vi "myRIO_BRig_Host_v0,31.vi"() -> ()   [LabVIEW 2014]
panel:
  out "output_L_or_R":i32
  out "element":u16
  out "error_LoadPrevSettings":errorcluster caption="error out"
  in  "LoadPrevSettings":bool
  out "graph_ai1":dbl(graph)
  out "graph_ai0":dbl(graph)
  in  "dataIn_maxTrialsDisplayed":i32 caption="Number of Trials Displayed\n( 0 = all trials )"
  out "error_TCP":errorcluster
  in  "stop":bool
  in  "colorIn_timeout":u32(colorbox)=7468543 caption="Choice Timeout"
  in  "colorIn_wrong/cue":u32(colorbox)=16728618 caption="Wrong Choice or\nLicked During Cue"
  in  "colorIn_reward":u32(colorbox)=5898088 caption="Reward"
  in  "colorIn_unknown":u32(colorbox)=16449331 caption="Unknown Trial Status"
  out "dataOut_plot":cluster{i32[], i32[]}[](graph)
  out "iTrial":i32
  out "iBlock":i32
  # "Exp Stats"
  # "Current Block Stats"
  # "Trials 2 Reward\n\nBad Trials\nPost Reward"
  # "Left Spout    Right Spout"
  # "Run Time\n\n   minutes    seconds"
  # "Average Block Stats"
  # "Trials 2 Reward\n\nBad Trials\nPost Reward"
  # "Left Spout    Right Spout"
  # "If you get ERROR 5 related to opening a file, press CONTINUE"
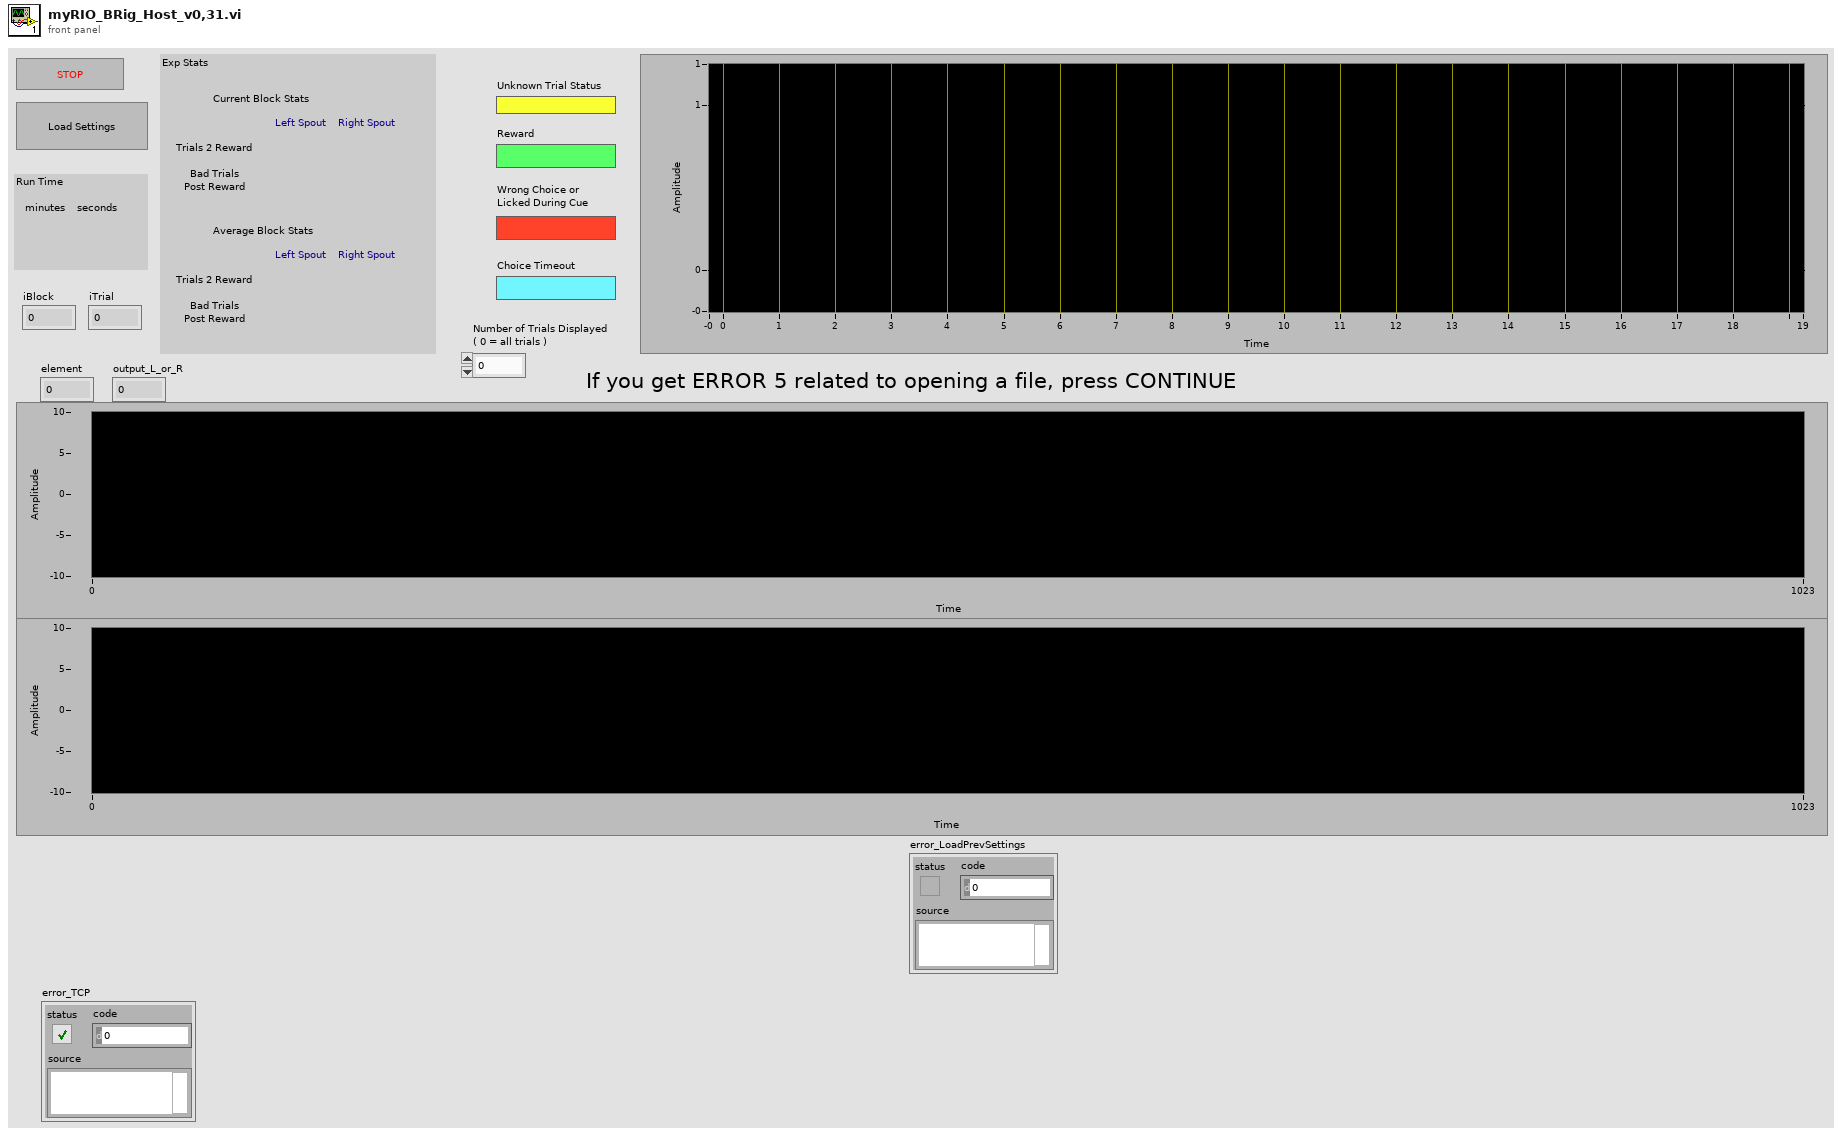
[diagram p1: front panel]
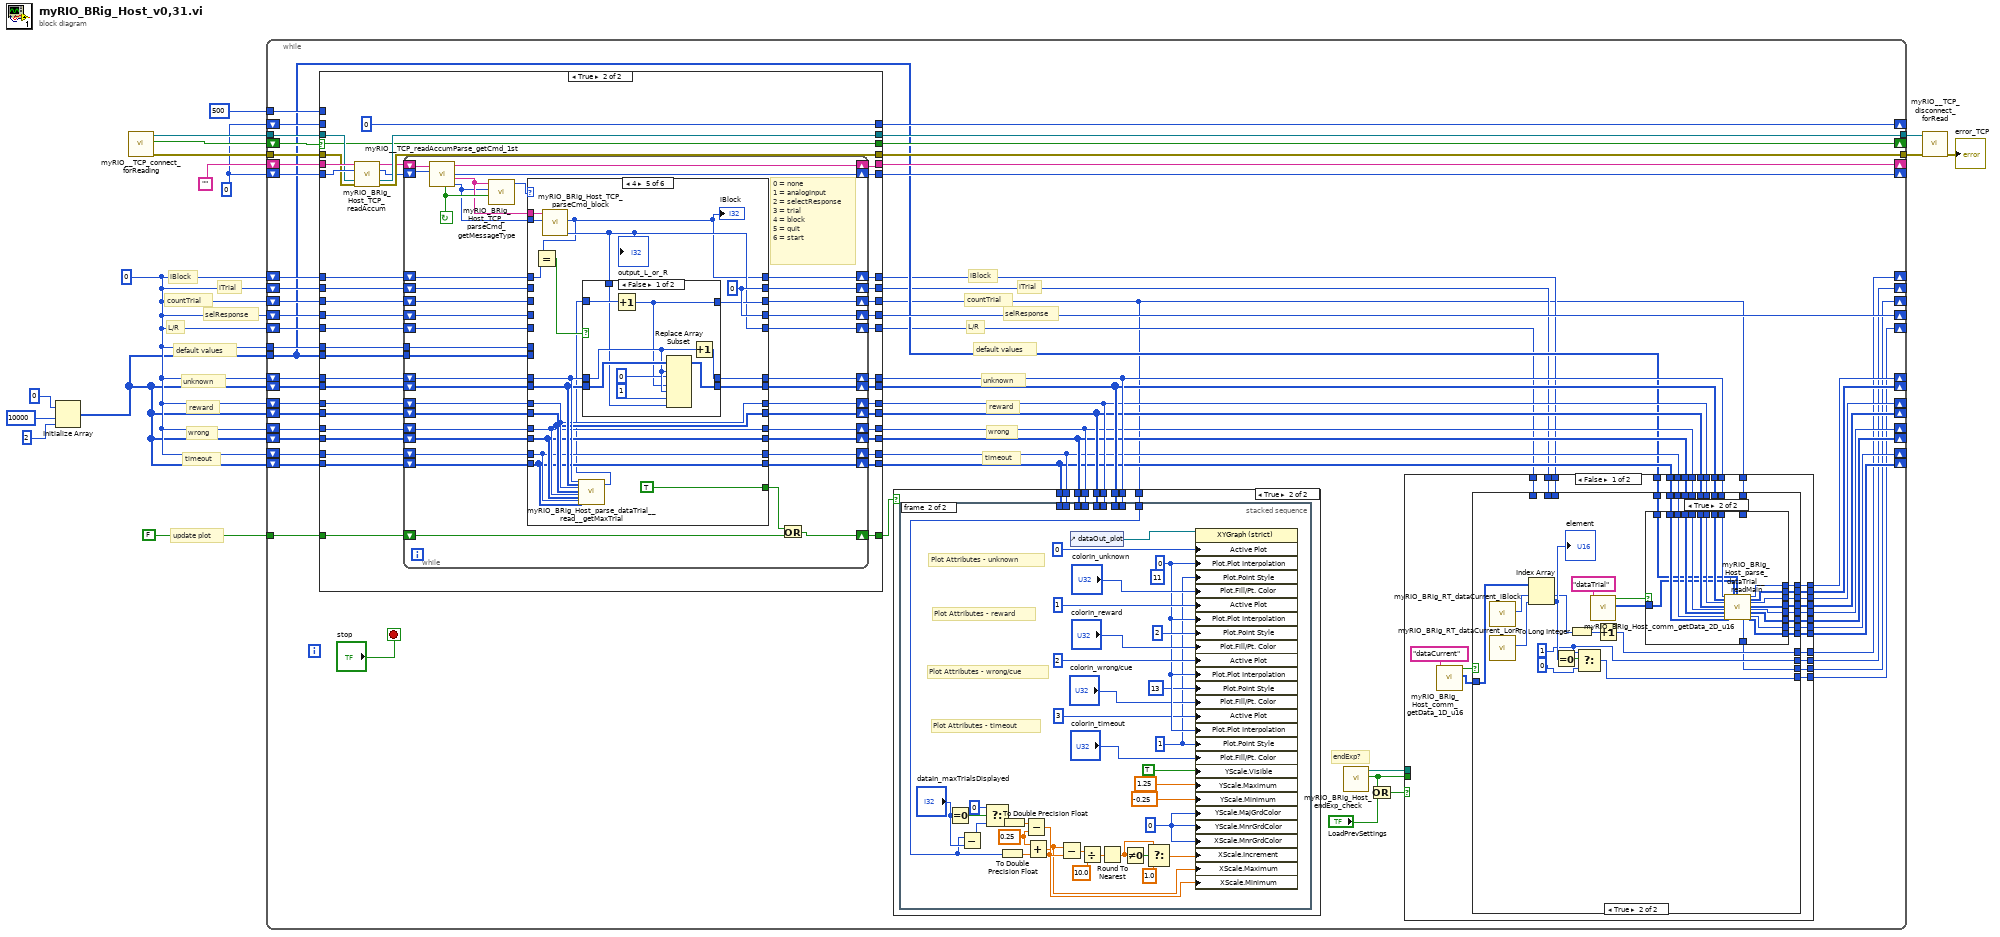
[diagram p0: block diagram]
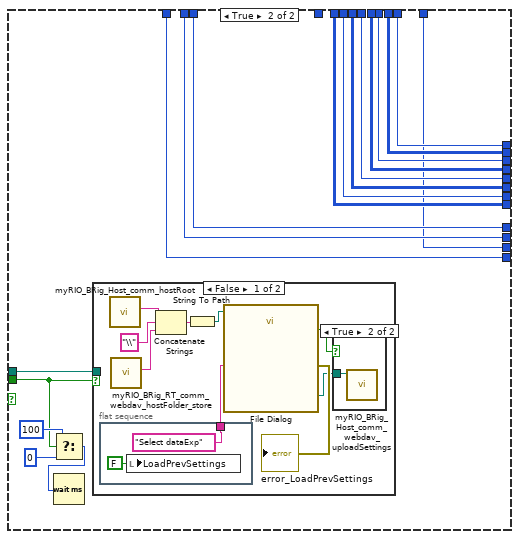
[diagram p4: hidden frame]
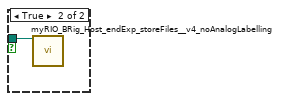
[diagram p6: hidden frame]
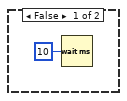
[diagram p7: hidden frame]
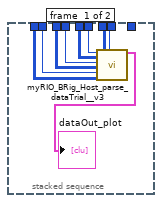
[diagram p8: hidden frame]
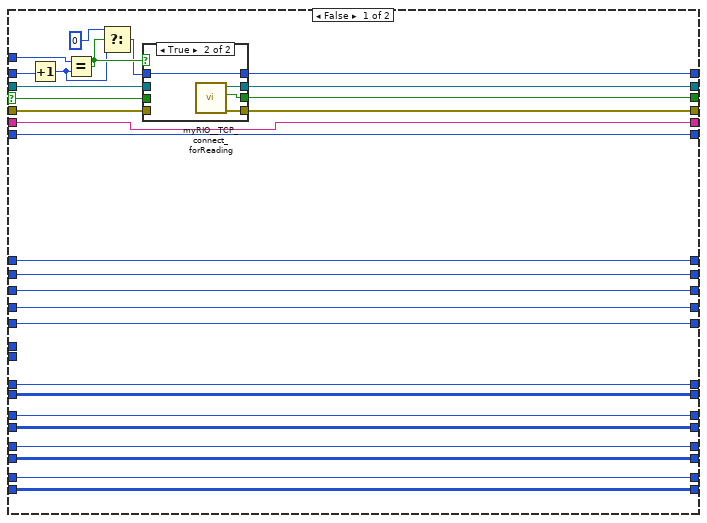
[diagram p9: hidden frame]
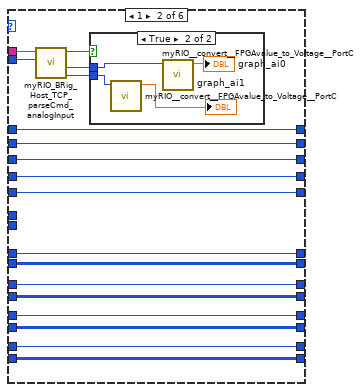
[diagram p12: hidden frame]
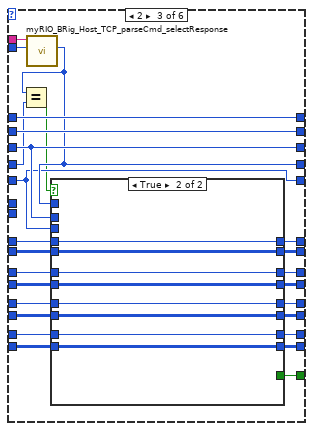
[diagram p14: hidden frame]
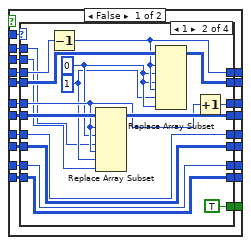
[diagram p15: hidden frame]
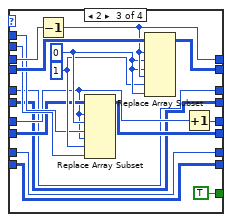
[diagram p17: hidden frame]
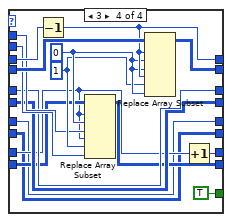
[diagram p18: hidden frame]
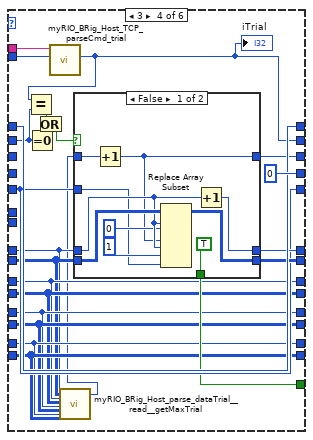
[diagram p19: hidden frame]
diagram:
  w2 = 0
  w11 = 0
  # "default values"
  # "update plot"
  # "timeout"
  # "wrong"
  # "reward"
  # "unknown"
  # "L/R"
  # "selResponse"
  # "countTrial"
  # "iBlock"
  # "iTrial"
  n1 = Initialize Array(0 ("element"), 10000 ("dimension size"), 2 ("dimension size")) -> (w1:i32[][])
  n2 = call "myRIO__TCP_connect_forReading.vi"() -> ("output_error"=w13:errorcluster, "output_connected"=w14:bool, "output_hTCP"=w15:refnum<k5>)  [unwired: 9 in]
  n3 = while {
    tunnel: w15 -> [w74]
    tunnel: w13 -> [w72]
    shift-right: [w65] -> _
    shift-left: w11 -> [w70]
    shift-right: [w66] -> _
    shift-left: "" -> [w71]
    shift-right: [w67] -> _
    shift-left: w14 -> [w73]
    shift-right: [w68] -> _
    shift-left: w11 -> [w75]
    tunnel: 500 ("y") -> [w69]
    shift-right: [w18] -> _
    shift-left: w2 -> [w64]
    shift-right: [w19] -> _
    shift-left: w2 -> [w63]
    shift-right: [w16] -> _
    shift-left: w2 -> [w62]
    shift-right: [w50] -> _
    shift-left: w2 -> [w61]
    shift-right: [w23] -> _
    shift-left: w2 -> [w60]
    shift-right: [w31] -> _
    shift-left: w2 -> [w59]
    shift-right: [w30] -> _
    shift-left: w1 -> [w58]
    shift-right: [w29] -> _
    shift-left: w2 -> [w57]
    shift-right: [w28] -> _
    shift-left: w1 -> [w56]
    shift-right: [w27] -> _
    shift-left: w2 -> [w55]
    shift-right: [w26] -> _
    shift-left: w1 -> [w54]
    shift-right: [w25] -> _
    shift-left: w2 -> [w53]
    shift-right: [w24] -> _
    shift-left: w1 -> [w52]
    tunnel: [w48] -> w5
    tunnel: [w47] -> w4
    tunnel: FALSE -> [w51]
    tunnel: w2 -> [w45]
    tunnel: w1 -> [w32]
    stop <- "stop" stop-if-true
    # "default values"
    # "timeout"
    # "wrong"
    # "reward"
    # "unknown"
    # "L/R"
    # "selResponse"
    # "countTrial"
    # "iBlock"
    # "iTrial"
    # "endExp?"
    n4 = case shown="True" w73 {
      selector: w73 -> [w283 w332]
      tunnel: w71 -> [w277 w338]
      tunnel: w70 -> [w278 w337]
      tunnel: [w277 w328] -> w66
      tunnel: [w278 w327] -> w65
      tunnel: w74 -> [w284 w336]
      tunnel: [w287 w335] -> w48
      tunnel: w72 -> [w282 w334]
      tunnel: [w286 w333] -> w47
      tunnel: [w285 w332] -> w67
      tunnel: w75 -> [w288 _]
      tunnel: [w276 0] -> w68
      tunnel: w69 -> [w275 _]
      tunnel: w64 -> [w274 w326]
      tunnel: w63 -> [w273 w325]
      tunnel: w62 -> [w272 w324]
      tunnel: w61 -> [w271 w323]
      tunnel: w60 -> [w270 w322]
      tunnel: w59 -> [w269 w321]
      tunnel: w58 -> [w268 w320]
      tunnel: w57 -> [w267 w319]
      tunnel: w56 -> [w266 w318]
      tunnel: w55 -> [w265 w317]
      tunnel: w54 -> [w264 w316]
      tunnel: w53 -> [w263 w315]
      tunnel: w52 -> [w262 w314]
      tunnel: w51 -> [_ w313]
      tunnel: [_ w312] -> w49
      tunnel: [w274 w311] -> w22
      tunnel: [w273 w310] -> w21
      tunnel: [w272 w309] -> w17
      tunnel: [w271 w308] -> w50
      tunnel: [w270 w307] -> w20
      tunnel: [w269 w306] -> w40
      tunnel: [w268 w305] -> w39
      tunnel: [w267 w304] -> w38
      tunnel: [w266 w303] -> w37
      tunnel: [w265 w302] -> w36
      tunnel: [w264 w301] -> w35
      tunnel: [w263 w300] -> w34
      tunnel: [w262 w299] -> w33
      tunnel: w45 -> [_ w298]
      tunnel: w32 -> [_ w297]
      frame False {
        n5 = Increment(x=w288) -> (x+1=w261:i32)
        n6 = Equal?(x=w275, y=w261) -> (x = y?=w281:bool)
        n7 = Select(t=0, s=w281, f=w261) -> (s? t:f=w279:i32)
        n8 = case shown="True" w281 {
          tunnel: w279 -> [w289 w293]
          tunnel: [w292 w296] -> w287
          tunnel: [w290 w295] -> w286
          tunnel: [w291 w294] -> w285
          tunnel: w284 -> [w292 _]
          tunnel: w283 -> [w291 _]
          tunnel: w282 -> [w290 _]
          tunnel: [w289 w293] -> w276
          frame False {
          }
          frame True {
            n9 = call "myRIO__TCP_connect_forReading.vi"() -> ("output_error"=w295:errorcluster, "output_connected"=w294:bool, "output_hTCP"=w296:refnum<k5>)  [unwired: 9 in]
          }
        }
      }
      frame True {
        n10 = call "myRIO_BRig_Host_TCP_readAccum.vi"("input_strAccum"=w338, "input_count"=w337, "input_handle_TCP"=w336, "input_error"=w334) -> ("output_strAccum"=w330:string, "output_count"=w329:i32, "output_handle_TCP"=w335:refnum<k5>, "output_error"=w333:errorcluster)  [unwired: 8 in]
        n11 = while {
          shift-right: [w375] -> w328
          shift-left: w330 -> [w377]
          shift-right: [w374] -> w327
          shift-left: w329 -> [w376]
          shift-right: [w366] -> w311
          shift-left: w326 -> [w369]
          shift-right: [w365] -> w310
          shift-left: w325 -> [w368]
          shift-right: [w364] -> w309
          shift-left: w324 -> [w367]
          shift-right: [w362] -> w308
          shift-left: w323 -> [w363]
          shift-right: [w360] -> w307
          shift-left: w322 -> [w361]
          shift-right: [w358] -> w306
          shift-left: w321 -> [w359]
          shift-right: [w356] -> w305
          shift-left: w320 -> [w357]
          shift-right: [w349] -> w304
          shift-left: w319 -> [w355]
          shift-right: [w348] -> w303
          shift-left: w318 -> [w354]
          shift-right: [w347] -> w302
          shift-left: w317 -> [w353]
          shift-right: [w346] -> w301
          shift-left: w316 -> [w352]
          shift-right: [w344] -> w299
          shift-left: w314 -> [w350]
          shift-right: [w345] -> w300
          shift-left: w315 -> [w351]
          shift-right: [w341] -> w312
          shift-left: w313 -> [w343]
          tunnel: w298 -> [w340]
          tunnel: w297 -> [w339]
          stop <- w373 continue-if-true
          # "0 = none\n1 = analogInput\n2 = selectResponse\n3 = trial\n4 = block\n5 = quit\n6 = start"
          n12 = call "myRIO__TCP_readAccumParse_getCmd_1st.vi"("input_count"=w376, "input_strAccum"=w377) -> ("output_countCmd"=w371:i32, "output_strCmd"=w372:string, "output_count"=w374:i32, "output_strAccum"=w375:string, "output_haveCmd"=w373:bool)  [unwired: 5 in]
          n13 = call "myRIO_BRig_Host_TCP_parseCmd_getMessageType.vi"("input_haveCmd"=w373, "input_countCmd"=w371, "input_strCmd"=w372) -> ("output_messageType"=w370:u8)  [unwired: 8 in]
          n14 = case shown="4" w370 {
            tunnel: w372 -> [_ w395 w437 w548 w580 w627]
            tunnel: w371 -> [_ w394 w436 w547 w579 _]
            tunnel: w369 -> [w390 w408 w438 w545 w573 w622]
            tunnel: w368 -> [w389 w407 w419 w539 _ w620]
            tunnel: w367 -> [w388 w406 w418 _ _ w619]
            tunnel: [w390 w408 w438 w545 w571 w621] -> w366
            tunnel: [w389 w407 w419 w538 w581 w616] -> w365
            tunnel: [w388 w406 w418 w542 w575 w615] -> w364
            tunnel: w363 -> [w387 w405 w416 _ _ w618]
            tunnel: [w387 w405 w415 0 ("output_iTrial_num") w581 w614] -> w362
            tunnel: w361 -> [w386 w404 w414 w541 _ w617]
            tunnel: [w386 w404 w414 w541 w574 w613] -> w360
            tunnel: w359 -> [w385 w403 w434 w527 w570 w612]
            tunnel: [w385 w403 w432 w544 w577 w604] -> w358
            tunnel: w357 -> [w384 w402 w435 w528 w569 w611]
            tunnel: [w384 w402 w433 w543 w578 w603] -> w356
            tunnel: w355 -> [w383 w401 w431 w529 w568 w610]
            tunnel: w354 -> [w382 w400 w430 w530 w567 w609]
            tunnel: w353 -> [w381 w399 w429 w531 w566 w608]
            tunnel: w352 -> [w380 w398 w428 w532 w565 w607]
            tunnel: w351 -> [w379 w397 w427 w533 w564 w606]
            tunnel: w350 -> [w378 w396 w426 w534 w563 w605]
            tunnel: [w383 w401 w420 w529 w568 w602] -> w349
            tunnel: [w382 w400 w421 w530 w567 w601] -> w348
            tunnel: [w381 w399 w422 w531 w566 w600] -> w347
            tunnel: [w380 w398 w423 w532 w565 w599] -> w346
            tunnel: [w379 w397 w424 w533 w564 w598] -> w345
            tunnel: [w378 w396 w425 w534 w563 w597] -> w344
            tunnel: [_ _ w417 w540 TRUE w594] -> w342
            tunnel: w340 -> [_ _ _ _ _ w596]
            tunnel: w339 -> [_ _ _ _ _ w595]
            frame 0, Default {
            }
            frame 1 {
              n15 = call "myRIO_BRig_Host_TCP_parseCmd_analogInput.vi"("input_countCmd"=w394, "input_strCmd"=w395) -> ("output_ai1"=w391:i32, "output_ai0"=w392:i32, "output_haveAnalogInput"=w393:bool)  [unwired: 7 in]
              n16 = case shown="True" w393 {
                tunnel: w392 -> [_ w412]
                tunnel: w391 -> [_ w410]
                frame False {
                }
                frame True {
                  n17 = call "myRIO__convert__FPGAvalue_to_Voltage__PortC.vi"("input_FPGAvalue_PortC"=w410) -> ("output_voltage"=→"graph_ai1":dbl)  [unwired: 10 in]
                  n18 = call "myRIO__convert__FPGAvalue_to_Voltage__PortC.vi"("input_FPGAvalue_PortC"=w412) -> ("output_voltage"=→"graph_ai0":dbl)  [unwired: 10 in]
                }
              }
            }
            frame 2 {
              n19 = call "myRIO_BRig_Host_TCP_parseCmd_selectResponse.vi"("input_countCmd"=w436, "input_strCmd"=w437) -> ("output_selectResponse_num"=w415:i32)  [unwired: 8 in, 1 out]
              n20 = Equal?(x=w415, y=w416) -> (x = y?=w413:bool)
              n21 = case shown="True" w413 {
                tunnel: w435 -> [w458 w524]
                tunnel: w434 -> [w457 w525]
                tunnel: [w456 w524] -> w433
                tunnel: [w455 w525] -> w432
                tunnel: w431 -> [w454 w523]
                tunnel: w430 -> [w453 w522]
                tunnel: w429 -> [w452 w521]
                tunnel: w428 -> [w451 w520]
                tunnel: w427 -> [w450 w519]
                tunnel: w426 -> [w449 w518]
                tunnel: [w448 w518] -> w425
                tunnel: [w447 w519] -> w424
                tunnel: [w446 w520] -> w423
                tunnel: [w445 w521] -> w422
                tunnel: [w444 w522] -> w421
                tunnel: [w443 w523] -> w420
                tunnel: w418 -> [w442 _]
                tunnel: [w441 _] -> w417
                tunnel: w415 -> [w440 _]
                tunnel: w414 -> [w439 _]
                frame False {
                  n22 = case shown="1" w440 {
                    tunnel: w458 -> [w465 w478 w498 w515]
                    tunnel: w457 -> [w466 w483 w500 w517]
                    tunnel: [w465 w477 w497 w514] -> w456
                    tunnel: [w466 w476 w496 w513] -> w455
                    tunnel: w454 -> [w459 w471 w484 w507]
                    tunnel: w453 -> [w460 w473 w485 w508]
                    tunnel: w452 -> [w461 w480 w488 w501]
                    tunnel: w451 -> [w462 w481 w489 w502]
                    tunnel: w450 -> [w463 w474 w494 w505]
                    tunnel: w449 -> [w464 w475 w495 w506]
                    tunnel: [w464 w475 w495 w503] -> w448
                    tunnel: [w463 w474 w494 w504] -> w447
                    tunnel: [w462 w481 w486 w502] -> w446
                    tunnel: [w461 w480 w487 w501] -> w445
                    tunnel: [w460 w472 w485 w508] -> w444
                    tunnel: [w459 w482 w484 w507] -> w443
                    tunnel: w442 -> [_ w468 w491 w510]
                    tunnel: [_ TRUE TRUE TRUE] -> w441
                    tunnel: w439 -> [_ w467 w490 w509]
                    frame 0, Default {
                    }
                    frame 1 {
                      w469 = 1 ("new element/subarray")
                      w470 = 0 ("new element/subarray")
                      n23 = Decrement(x=w483) -> (x-1=w476:i32)
                      n24 = Replace Array Subset(array=w473, new element #1=w468, index (row) #1=w471, index (col) #1=w470, new element #2=w467, index (row) #2=w471, index (col) #2=w469) -> (w472:i32[][])
                      n25 = Replace Array Subset(array=w478, new element #1=w470, index (row) #1=w476, index (col) #1=w470, new element #2=w470, index (row) #2=w476, index (col) #2=w469) -> (w477:i32[][])
                      n26 = Increment(x=w471) -> (x+1=w482:i32)
                    }
                    frame 2 {
                      w492 = 1 ("new element/subarray")
                      w493 = 0 ("new element/subarray")
                      n27 = Decrement(x=w500) -> (x-1=w496:i32)
                      n28 = Replace Array Subset(array=w489, new element #1=w491, index (row) #1=w488, index (col) #1=w493, new element #2=w490, index (row) #2=w488, index (col) #2=w492) -> (w486:i32[][])
                      n29 = Replace Array Subset(array=w498, new element #1=w493, index (row) #1=w496, index (col) #1=w493, new element #2=w493, index (row) #2=w496, index (col) #2=w492) -> (w497:i32[][])
                      n30 = Increment(x=w488) -> (x+1=w487:i32)
                    }
                    frame 3 {
                      w511 = 1 ("new element/subarray")
                      w512 = 0 ("new element/subarray")
                      n31 = Decrement(x=w517) -> (x-1=w513:i32)
                      n32 = Replace Array Subset(array=w506, new element #1=w510, index (row) #1=w505, index (col) #1=w512, new element #2=w509, index (row) #2=w505, index (col) #2=w511) -> (w503:i32[][])
                      n33 = Replace Array Subset(array=w515, new element #1=w512, index (row) #1=w513, index (col) #1=w512, new element #2=w512, index (row) #2=w513, index (col) #2=w511) -> (w514:i32[][])
                      n34 = Increment(x=w505) -> (x+1=w504:i32)
                    }
                  }
                }
                frame True {
                }
              }
            }
            frame 3 {
              n35 = Equal To 0?(x=w539) -> (x = 0?=w536:bool)
              n36 = call "myRIO_BRig_Host_TCP_parseCmd_trial.vi"("input_countCmd"=w547, "input_strCmd"=w548) -> ("output_iTrial_num"=w538:i32)  [unwired: 8 in, 1 out]
              "iTrial" <- w538
              n37 = Equal?(x=w538, y=w539) -> (x = y?=w537:bool)
              n38 = Or(x=w537, y=w536) -> (x .or. y?=w535:bool)
              n39 = call "myRIO_BRig_Host_parse_dataTrial__read__getMaxTrial.vi"("input_idxUnknown"=w527, "input_arrayUnknown"=w528, "input_idxReward"=w529, "input_arrayReward"=w530, "input_idxWrong"=w531, "input_arrayWrong"=w532, "input_idxTimeout"=w533, "input_arrayTimeout"=w534) -> ("output_maxTrial"=w526:i32)  [unwired: 19 in]
              n40 = case shown="False" w535 {
                tunnel: w527 -> [w557 w561]
                tunnel: w528 -> [w558 w560]
                tunnel: w526 -> [w552 w559]
                tunnel: [w556 w561] -> w544
                tunnel: [w555 w560] -> w543
                tunnel: [w551 w559] -> w542
                tunnel: w541 -> [w550 _]
                tunnel: [TRUE _] -> w540
                frame False {
                  n41 = Increment(x=w552) -> (x+1=w551:i32)
                  n42 = Replace Array Subset(array=w558, new element #1=w551, index (row) #1=w557, index (col) #1=0 ("new element/subarray"), new element #2=w550, index (row) #2=w557, index (col) #2=1 ("new element/subarray")) -> (w555:i32[][])
                  n43 = Increment(x=w557) -> (x+1=w556:i32)
                }
                frame True {
                }
              }
            }
            frame 4 {
              w581 = 0 ("output_iTrial_num")
              n44 = call "myRIO_BRig_Host_TCP_parseCmd_block.vi"("input_countCmd"=w579, "input_strCmd"=w580) -> ("output_L_or_R"=w574:i32, "output_iBlock_num"=w571:i32)  [unwired: 7 in, 1 out]
              "iBlock" <- w571
              "output_L_or_R" <- w574
              n45 = Equal?(x=w571, y=w573) -> (x = y?=w572:bool)
              n46 = call "myRIO_BRig_Host_parse_dataTrial__read__getMaxTrial.vi"("input_idxUnknown"=w570, "input_arrayUnknown"=w569, "input_idxReward"=w568, "input_arrayReward"=w567, "input_idxWrong"=w566, "input_arrayWrong"=w565, "input_idxTimeout"=w564, "input_arrayTimeout"=w563) -> ("output_maxTrial"=w562:i32)  [unwired: 19 in]
              n47 = case shown="False" w572 {
                tunnel: w562 -> [w590 w591]
                tunnel: w569 -> [w589 w592]
                tunnel: [w588 w592] -> w578
                tunnel: [w587 w593] -> w577
                tunnel: w570 -> [w586 w593]
                tunnel: w574 -> [w583 _]
                tunnel: [w582 w591] -> w575
                frame False {
                  n48 = Increment(x=w590) -> (x+1=w582:i32)
                  n49 = Replace Array Subset(array=w589, new element #1=w582, index (row) #1=w586, index (col) #1=0 ("new element/subarray"), new element #2=w583, index (row) #2=w586, index (col) #2=1 ("new element/subarray")) -> (w588:i32[][])
                  n50 = Increment(x=w586) -> (x+1=w587:i32)
                }
                frame True {
                }
              }
            }
            frame 6 {
              n51 = String Subset(string=w627, offset (0)=2, length (rest)=1 ("length (rest)")) -> (substring=w624:string)
              n52 = Equal?(x=w624, y="e") -> (x = y?=w594:bool)
              n53 = case shown="True" w594 {
                tunnel: w622 -> [w640 _]
                tunnel: [w640 w642] -> w621
                tunnel: w620 -> [w639 _]
                tunnel: w619 -> [w638 _]
                tunnel: w618 -> [w637 _]
                tunnel: w617 -> [w636 _]
                tunnel: [w639 w642] -> w616
                tunnel: [w638 w642] -> w615
                tunnel: [w637 w642] -> w614
                tunnel: [w636 w642] -> w613
                tunnel: w612 -> [w635 _]
                tunnel: w611 -> [w634 _]
                tunnel: w610 -> [w633 _]
                tunnel: w609 -> [w632 _]
                tunnel: w608 -> [w631 _]
                tunnel: w607 -> [w630 _]
                tunnel: w606 -> [w629 _]
                tunnel: w605 -> [w628 _]
                tunnel: [w635 w642] -> w604
                tunnel: [w634 w641] -> w603
                tunnel: [w633 w642] -> w602
                tunnel: [w632 w641] -> w601
                tunnel: [w631 w642] -> w600
                tunnel: [w630 w641] -> w599
                tunnel: [w629 w642] -> w598
                tunnel: [w628 w641] -> w597
                tunnel: w596 -> [_ w642]
                tunnel: w595 -> [_ w641]
                frame False {
                }
                frame True {
                }
              }
            }
          }
          n54 = Or(x=w342, y=w343) -> (x .or. y?=w341:bool)
        }
      }
    }
    n55 = case shown="True" w49 {
      tunnel: w33 -> [_ w216]
      tunnel: w34 -> [_ w215]
      tunnel: w35 -> [_ w214]
      tunnel: w36 -> [_ w213]
      tunnel: w37 -> [_ w212]
      tunnel: w38 -> [_ w211]
      tunnel: w39 -> [_ w210]
      tunnel: w40 -> [_ w209]
      tunnel: w17 -> [_ w208]
      frame False {
        n56 = Wait (ms)(milliseconds to wait=u32 10) -> ()  [unwired: 1 out]
      }
      frame True {
        n57 = stacked-sequence {
          tunnel: w216 -> [w225 _]
          tunnel: w215 -> [w224 _]
          tunnel: w214 -> [w223 _]
          tunnel: w213 -> [w222 _]
          tunnel: w212 -> [w221 _]
          tunnel: w211 -> [w220 _]
          tunnel: w210 -> [w219 _]
          tunnel: w209 -> [w218 _]
          tunnel: w208 -> [_ w234]
          frame #0 {
            n58 = call "myRIO_BRig_Host_parse_dataTrial__v3.vi"("input_idxReward"=w220, "input_arrayReward"=w221, "input_idxWrong"=w222, "input_arrayWrong"=w223, "input_idxTimeout"=w224, "input_arrayTimeout"=w225, "input_arrayUnknown"=w219, "input_idxUnknown"=w218) -> ("output_plotData"=→"dataOut_plot":cluster{i32[], i32[]}[])  [unwired: 11 in]
          }
          frame #1 {
            w230 = u32 0 ("Y Scale.Grid Colors:Major Color")
            w238 = 0.25 ("y")
            w227 = u8 1 ("Plot.Point Style")
            (unwired) u8 11 ("Plot.Point Style")
            w254 = u8 0 ("Plot.Plot Interpolation")
            # "Plot Attributes - timeout"
            # "Plot Attributes - wrong/cue"
            # "Plot Attributes - reward"
            # "Plot Attributes - unknown"
            n59 = Equal To 0?(x="dataIn_maxTrialsDisplayed") -> (x = 0?=w235:bool)
            n60 = Subtract(x=w234, y="dataIn_maxTrialsDisplayed") -> (x-y=w236:i32)
            n61 = Select(t=0, s=w235, f=w236) -> (s? t:f=w241:i32)
            n62 = To Double Precision Float(number=w234) -> (double precision float=w239:dbl)
            n63 = To Double Precision Float(number=w241) -> (double precision float=w240:dbl)
            n64 = Subtract(x=w240, y=w238) -> (x-y=w228:dbl)
            n65 = Add(x=w238, y=w239) -> (x+y=w226:dbl)
            n66 = Subtract(x=w226, y=w228) -> (x-y=w242:dbl)
            n67 = control-ref of="dataOut_plot"() -> (w249:refnum<vi>)
            n68 = Divide(x=w242, y=10.0) -> (x/y=w244:dbl)
            n69 = Round To Nearest(number=w244) -> (nearest integer value=w246:dbl)
            n70 = Not Equal To 0?(x=w246) -> (x != 0?=w245:bool)
            n71 = Select(t=w246, s=w245, f=1.0) -> (s? t:f=w229:dbl)
            n72 = property on="Property Node" class="XYGraph (strict)"(reference=w249, "Active Plot"=u32 0, "Plot.Plot Interpolation"=w254, "Plot.Point Style"=w227, "Plot.Fill/Pt. Color"="colorIn_unknown", "Active Plot"=u32 1, "Plot.Plot Interpolation"=w254, "Plot.Point Style"=u8 2, "Plot.Fill/Pt. Color"="colorIn_reward", "Active Plot"=u32 2, "Plot.Plot Interpolation"=w254, "Plot.Point Style"=u8 13, "Plot.Fill/Pt. Color"="colorIn_wrong/cue", "Active Plot"=u32 3, "Plot.Plot Interpolation"=w254, "Plot.Point Style"=w227, "Plot.Fill/Pt. Color"="colorIn_timeout", "YScale.Visible"=TRUE ("Y Scale.Visible"), "YScale.Maximum"=1.25 ("Y Scale.Range:Maximum"), "YScale.Minimum"=-0.25 ("Y Scale.Range:Minimum"), "YScale.MajGrdColor"=w230, "YScale.MnrGrdColor"=w230, "XScale.MnrGrdColor"=w230, "XScale.Increment"=w229, "XScale.Maximum"=w226, "XScale.Minimum"=w228) -> ()  [unwired: 1 in, 2 out]
          }
        }
      }
    }
    n73 = call "myRIO_BRig_Host_endExp_check.vi"() -> ("output_IendExp"=w42:bool, "output_filePath_expExp"=w41:path)  [unwired: 10 in]
    n74 = Or(x=w42, y="LoadPrevSettings") -> (x .or. y?=w43:bool)
    n75 = case shown="False" w43 {
      tunnel: w42 -> [_ w190]
      tunnel: w41 -> [_ w189]
      tunnel: [w100 w188] -> w31
      tunnel: [w99 w187] -> w30
      tunnel: [w98 w186] -> w29
      tunnel: [w97 w185] -> w28
      tunnel: [w96 w184] -> w27
      tunnel: [w95 w183] -> w26
      tunnel: [w94 w182] -> w25
      tunnel: [w93 w181] -> w24
      tunnel: w40 -> [w92 w188]
      tunnel: w39 -> [w91 w187]
      tunnel: w38 -> [w90 w186]
      tunnel: w37 -> [w89 w185]
      tunnel: w36 -> [w88 w184]
      tunnel: w35 -> [w87 w183]
      tunnel: w34 -> [w86 w182]
      tunnel: w33 -> [w85 w181]
      tunnel: w32 -> [w84 _]
      tunnel: [w83 w178] -> w23
      tunnel: [w82 w179] -> w19
      tunnel: [w81 w180] -> w18
      tunnel: w22 -> [w80 w180]
      tunnel: w21 -> [w79 w179]
      tunnel: w20 -> [w78 w178]
      tunnel: [w77 w177] -> w16
      tunnel: w17 -> [w76 w177]
      frame False {
        n76 = call "myRIO_BRig_Host_comm_getData_1D_u16.vi"("input_fileName"="dataCurrent") -> ("output_data_1D"=w101:u16[], "output_I_data"=w102:bool)  [unwired: 9 in]
        n77 = case shown="True" w102 {
          tunnel: w101 -> [_ w148]
          tunnel: [w115 w143] -> w100
          tunnel: [w114 w142] -> w99
          tunnel: [w113 w141] -> w98
          tunnel: [w112 w140] -> w97
          tunnel: [w111 w139] -> w96
          tunnel: [w110 w138] -> w95
          tunnel: [w109 w137] -> w94
          tunnel: [w108 w136] -> w93
          tunnel: w92 -> [w115 w135]
          tunnel: w91 -> [w114 w134]
          tunnel: w90 -> [w113 w133]
          tunnel: w89 -> [w112 w132]
          tunnel: w88 -> [w111 w131]
          tunnel: w87 -> [w110 w130]
          tunnel: w86 -> [w109 w129]
          tunnel: w85 -> [w108 w128]
          tunnel: w84 -> [_ w127]
          tunnel: [w105 w123] -> w83
          tunnel: [w106 w122] -> w82
          tunnel: [w107 w118] -> w81
          tunnel: w80 -> [w107 _]
          tunnel: w79 -> [w106 _]
          tunnel: w78 -> [w105 _]
          tunnel: [w104 w117] -> w77
          tunnel: w76 -> [w104 w116]
          frame False {
          }
          frame True {
            w122 = 1
            n78 = call "myRIO_BRig_RT_dataCurrent_iBlock.vi"() -> ("output_iBlock"=w121:i32)  [unwired: 11 in]
            n79 = call "myRIO_BRig_RT_dataCurrent_LorR.vi"() -> ("output_LorR"=w144:i32)  [unwired: 11 in]
            n80 = Index Array(array=w148, index #1=w121, index #2=w144) -> (element #1=w120:u16, element #2=w126:u16)
            "element" <- w126
            n81 = Equal To 0?(x=w126) -> (x = 0?=w125:bool)
            n82 = To Long Integer(number=w120) -> (32bit integer=w119:i32)
            n83 = Select(t=w122, s=w125, f=0) -> (s? t:f=w123:i32)
            n84 = call "myRIO_BRig_Host_comm_getData_2D_u16.vi"("input_fileName"="dataTrial") -> ("output_data_2D"=w145:u16[][], "output_I_data"=w146:bool)  [unwired: 9 in]
            n85 = Increment(x=w119) -> (x+1=w118:i32)
            n86 = case shown="True" w146 {
              tunnel: w145 -> [_ w168]
              tunnel: [w155 w164] -> w141
              tunnel: [w154 w163] -> w140
              tunnel: [w156 w165] -> w142
              tunnel: [w157 w166] -> w143
              tunnel: [w153 w162] -> w139
              tunnel: [w152 w161] -> w138
              tunnel: [w151 w160] -> w137
              tunnel: [w150 w159] -> w136
              tunnel: w127 -> [_ w167]
              tunnel: w135 -> [w157 w176]
              tunnel: w134 -> [w156 w175]
              tunnel: w133 -> [w155 w174]
              tunnel: w132 -> [w154 w173]
              tunnel: w131 -> [w153 w172]
              tunnel: w130 -> [w152 w171]
              tunnel: w129 -> [w151 w170]
              tunnel: w128 -> [w150 w169]
              tunnel: [w149 w158] -> w117
              tunnel: w116 -> [w149 _]
              frame False {
              }
              frame True {
                n87 = call "myRIO_BRig_Host_parse_dataTrial__readMain.vi"("input_idxUnknown"=w176, "input_arrayUnknown"=w175, "input_idxReward"=w174, "input_arrayReward"=w173, "input_idxWrong"=w172, "input_arrayWrong"=w171, "input_idxTimeout"=w170, "input_arrayTimeout"=w169, "arrayIn_dataTrial"=w168, "arrayIn_empty"=w167) -> ("output_countTrial"=w158:i32, "output_idxUnknown"=w166:i32, "output_arrayUnknown"=w165:i32[][], "output_idxReward"=w164:i32, "output_arrayReward"=w163:i32[][], "output_idxWrong"=w162:i32, "output_arrayWrong"=w161:i32[][], "output_idxTimeout"=w160:i32, "output_arrayTimeout"=w159:i32[][])  [unwired: 9 in]
              }
            }
          }
        }
      }
      frame True {
        n88 = Select(t=u32 100 ("milliseconds to wait"), s=w190, f=u32 0 ("milliseconds to wait")) -> (s? t:f=w192:u32)
        n89 = Wait (ms)(milliseconds to wait=w192) -> ()  [unwired: 1 out]
        n90 = case shown="False" w190 {
          tunnel: w189 -> [_ w206]
          frame False {
            n91 = flat-sequence {
              tunnel: ["Select dataExp" ("prompt")] -> w197
              frame #0 {
                n92 = local write "LoadPrevSettings"(FALSE ("LoadPrevSettings")) -> ()
              }
            }
            n93 = call "myRIO_BRig_Host_comm_hostRoot.vi"() -> ("output_hostRoot"=w199:string)  [unwired: 11 in]
            n94 = call "myRIO_BRig_RT_comm_webdav_hostFolder_store.vi"() -> ("output_HostFolder"=w201:string)  [unwired: 11 in]
            n95 = Concatenate Strings(w199, "\\" ("string"), w201) -> (w202:string)
            n96 = String To Path(string=w202) -> (path=w198:path)
            n97 = call "File Dialog"("start path"=w198, "prompt"=w197) -> ("selected path"=w194:path, "exists"=w195:bool, "error out"=→"error_LoadPrevSettings":errorcluster)  [unwired: 10 in, 1 out]
            n98 = case shown="True" w195 {
              tunnel: w194 -> [_ w203]
              frame False {
              }
              frame True {
                n99 = call "myRIO_BRig_Host_comm_webdav_uploadSettings.vi"("input_filePath"=w203) -> ()  [unwired: 11 in]
              }
            }
          }
          frame True {
            n100 = call "myRIO_BRig_Host_endExp_storeFiles__v4_noAnalogLabelling.vi"("input_filePath"=w206) -> ()  [unwired: 15 in]
          }
        }
      }
    }
  }
  n101 = call "myRIO__TCP_disconnect_forRead.vi"("input_error"=w4, "input_hTCP"=w5) -> ("output_error"=→"error_TCP":errorcluster)  [unwired: 9 in]
